vi "Test Instrument Remote API.vi"   [LabVIEW 2019]
uses:
  <vilib>/JKI/JKI SMO/SMO/Typedefs/SMOState --Enum.ctl
  lvsrc/Framework-Template/SMOs/Instrument.Framework-Template/Instrument.Framework-Template.lvclass
  C:/Users/patrick/Documents/GitHub/Instrument-Framework/lvsrc/Instrument/Instrument.lvclass
  C:/Program Files (x86)/National Instruments/LabVIEW 2019/vi.lib/JKI/JKI SMO/SMO/SMO.lvclass
  <vilib>/addons/_JKI Toolkits/Caraya/classes/Assert/Assert Equal Value and Type_Variant.vi
  <vilib>/addons/_JKI Toolkits/Caraya/classes/Assert/Assert Not Error.vi
  lvsrc/Framework/Instrument/Instrument.lvclass
  2883ed84-2e87-409c-95c0-cbb5fa801e98.vi
  <vilib>/JKI/JKI SMO/SMO/SMO.lvclass
  <vilib>/addons/_JKI Toolkits/Caraya/classes/Assert/Assert.lvclass
  <vilib>/addons/_JKI Toolkits/Caraya/classes/Test/Test.lvclass
types:
  T1 = typedef "SMO.lvclass/SMOState --Enum.ctl" = enum16{"unknown", "Created", "Started", "Stopped"}
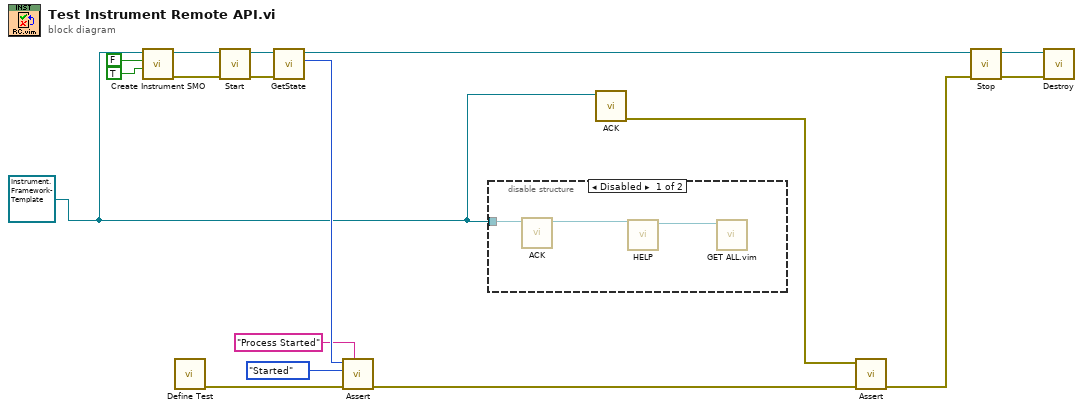
[diagram p0: block diagram]
diagram:
  w1 = refnum<class "Instrument.Framework-Template.lvclass"> refnum ("Instrument.Framework-Template.lvclass")
  n1 = call "Create Instrument SMO.vi"("Debug Mode? [F]"=TRUE, "Configuration Window? [T]"=FALSE, "Instrument in"=w1) -> ("error out"=w15:errorcluster, "Instrument out"=w16:refnum<class "Instrument.Framework-Template.lvclass">)  [unwired: 7 in]
  n2 = call <vilib>:"Define Test.vi"() -> ("error out"=w7:errorcluster)  [unwired: 10 in, 1 out]
  n3 = call <vilib>:"Start.vi"("error in (no error)"=w15, "SMO"=w16) -> ("error out"=w12:errorcluster, "SMO out"=w11:refnum<class "Instrument.Framework-Template.lvclass">)  [unwired: 8 in]
  n4 = call <vilib>:"GetState.vi"("error in (no error)"=w12, "SMO"=w11) -> ("SMO State"=w10:T1, "SMO out"=w8:refnum<class "Instrument.Framework-Template.lvclass">)  [unwired: 7 in, 1 out]
  n5 = call-poly <vilib>:"Assert.vi"("Label"="Process Started", "error in (no error)"=w7, "Y"=SMOState_--Enum."Started" ("SMO State"), "X"=w10) -> ("error out"=w5:errorcluster)  [unwired: 6 in, 1 out]
  n6 = disable-structure shown="Disabled" {
    disable-tunnel: w1 -> [w18 _]
    frame Disabled {
      n7 = call "ACK.vi"("Instrument in"=w18) -> ("Instrument out"=w20:refnum<class "Instrument.Framework-Template.lvclass">)  [unwired: 8 in, 2 out]
      n8 = call "HELP.vi"("Instrument in"=w20) -> ("Instrument in"=w19:refnum<class "Instrument.Framework-Template.lvclass">)  [unwired: 8 in, 2 out]
      n9 = call "GET ALL.vim"("Instrument in"=w19) -> ()  [unwired: 8 in, 3 out]
    }
    frame Enabled {
    }
  }
  n10 = call "ACK.vi"("Instrument in"=w1) -> ("error out"=w4:errorcluster)  [unwired: 8 in, 2 out]
  n11 = call-poly <vilib>:"Assert.vi"("error in (no error)"=w5, "Not Error?"=w4) -> ("error out"=w3:errorcluster)  [unwired: 8 in, 1 out]
  n12 = call <vilib>:"Stop.vi"("error in (no error)"=w3, "SMO"=w8) -> ("error out"=w13:errorcluster, "SMO out"=w14:refnum<class "Instrument.Framework-Template.lvclass">)  [unwired: 8 in]
  n13 = call <vilib>:"Destroy.vi"("error in (no error)"=w13, "SMO"=w14) -> ()  [unwired: 9 in, 1 out]
